vi "Main.vi"(11 "Module Admin":refnum<class "Delacor_lib_QMH_Module Admin.lvclass">) -> ()   [LabVIEW 2019, in "UI.lvlib"]
doc: "This template is based off of the Queued Message Handler design pattern and the Queued Message Handler project template that ships with LabVIEW.\n\nThe main difference is that the queue is private to this module and communication between modules is performed via Broadcast and Request events.\n\nRequest events are wrapped in public API methods and are handled in the Event Handling Loop (EHL) of this VI. Any module can register for Broadcast events sent by this module. The EHL generates messages based on user interface actions.\n\nThe Message Handling Loop (MHL) processes messages generated by the EHL, or by other messages. The messages are string values, so new messages can be added easily to the Message Cases case structure in the MHL. Each message cluster can also provide an optional value for Message Data, which is a variant that can be converted to whatever message-specific data is required.\n_____\nBased on Delacor QMH Project Template 5.0.0.82."
uses:
  UI.lvlib
  <vilib>/Delacor/Delacor QMH/Libraries/Module Admin_class/Delacor_lib_QMH_Module Admin.lvclass
  Module Data--cluster.ctl
  Stop Argument--cluster.ctl
  <vilib>/Delacor/Delacor QMH/Libraries/Message Queue_class/Delacor_lib_QMH_Message Queue.lvclass/Delacor_lib_QMH_Message Queue.ctl
  <vilib>/Delacor/Delacor QMH/Libraries/Module Admin_class/Delacor_lib_QMH_Module Admin.lvclass/Delacor_lib_QMH_Module Admin.ctl
  <vilib>/Utility/miscctls.llb/LVPointTypeDef.ctl
  <vilib>/Delacor/Delacor QMH/Libraries/Message Queue_class/Delacor_lib_QMH_Enqueue Message (Single).vi
  <vilib>/Delacor/Delacor QMH/Libraries/Module Admin_class/Delacor_lib_QMH_Get External Launch.vi
  <vilib>/Utility/error.llb/Error Cluster From Error Code.vi
  <vilib>/ErrorRing/Error Ring.xnode
  <vilib>/Delacor/Delacor QMH/Libraries/Message Queue_class/Delacor_lib_QMH_Message Queue.lvclass
  LabVIEW Data/DQMH Module Templates/Source/Luis/Modulo w HL(with Helper Loop)/Modulo w HL(with Helper Loop).lvlib
panel:
  in  "Stop Acq":bool
  in  "Start Acq":bool
  out "error out":errorcluster
  out "Status":string
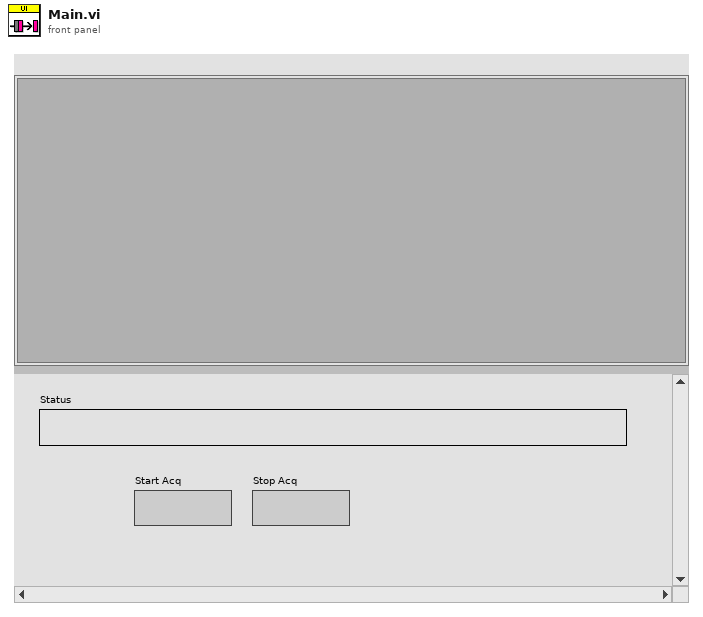
[diagram p1: front panel]
types:
  T1 = typedef "UI.lvlib/Request Events--cluster.ctl" = cluster{"Stop Module":refnum<user-event>, "Show Panel":refnum<user-event>, "Hide Panel":refnum<user-event>, "Get Module Execution Status":refnum<user-event>, "Show Diagram":refnum<user-event>}
  T2 = typedef "Aquisition.lvlib/Broadcast Events--cluster.ctl" = cluster{"Module Did Init":refnum<user-event>, "Status Updated":refnum<user-event>, "Error Reported":refnum<user-event>, "Module Did Stop":refnum<user-event>, "Update Module Execution Status":refnum<user-event>}
  T3 = typedef "UI.lvlib/Module Data--cluster.ctl" = cluster{"Status":string}
  T4 = enum32{"invalid lock state", "Not Locked", "Locked (No Password)", "Password-protected"}
  T5 = typedef "UI.lvlib/Stop Argument--cluster.ctl" = cluster{"Origin":string, "Exit via Stop Module Req?":bool, "Wait for Module to stop?":bool}
  T6 = enum32{"Invalid", "Standard", "Closed", "Hidden", "Minimized", "Maximized"}
  T7 = typedef "LVPointTypeDef.ctl" = cluster{"Horizontal":i16, "Vertical":i16}
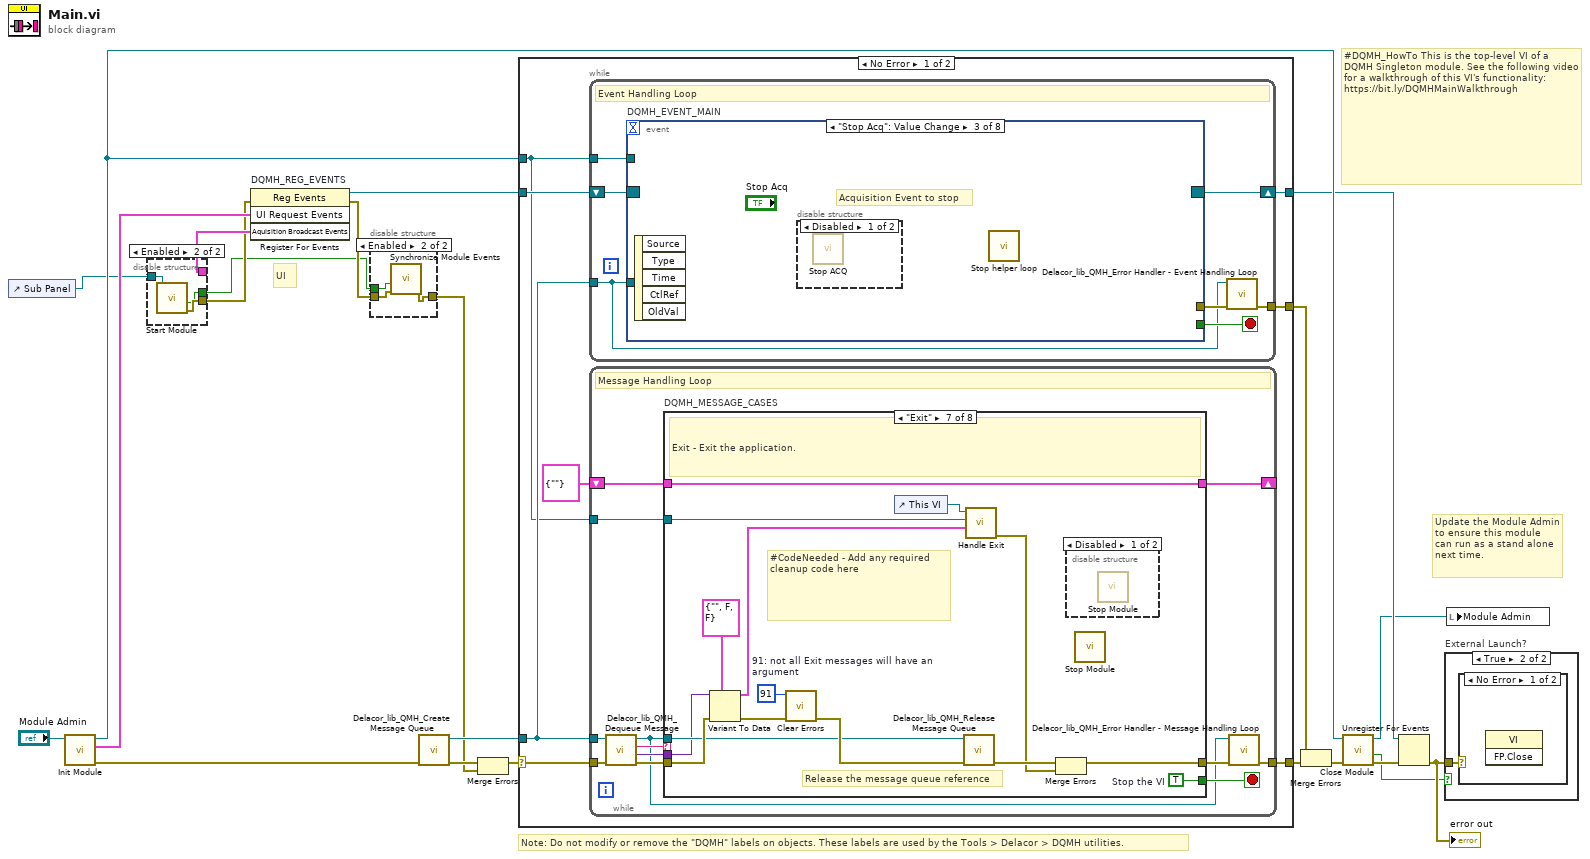
[diagram p0: block diagram]
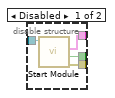
[diagram p2: hidden frame]
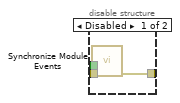
[diagram p3: hidden frame]
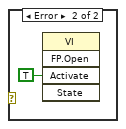
[diagram p5: hidden frame]
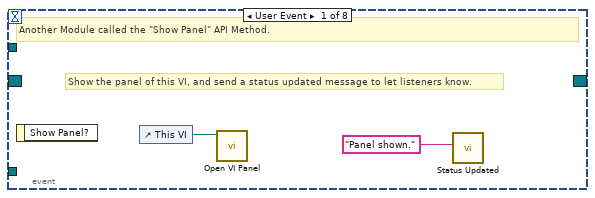
[diagram p6: hidden frame]
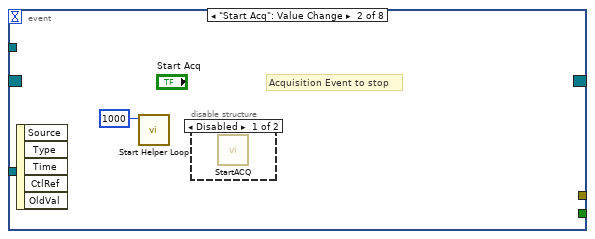
[diagram p7: hidden frame]
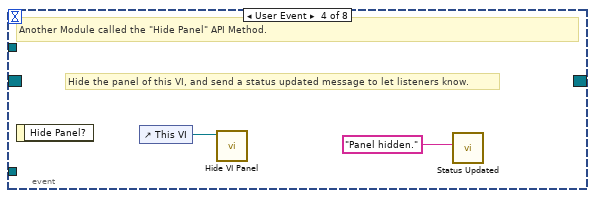
[diagram p10: hidden frame]
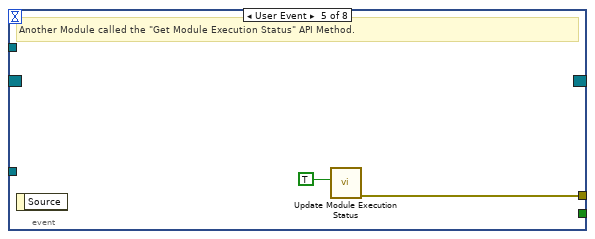
[diagram p11: hidden frame]
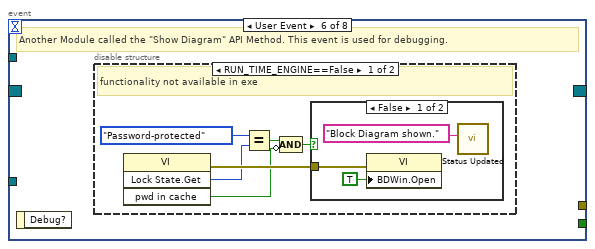
[diagram p12: hidden frame]
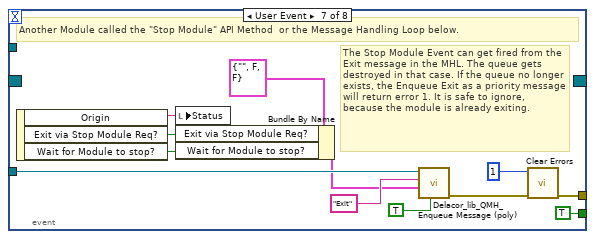
[diagram p15: hidden frame]
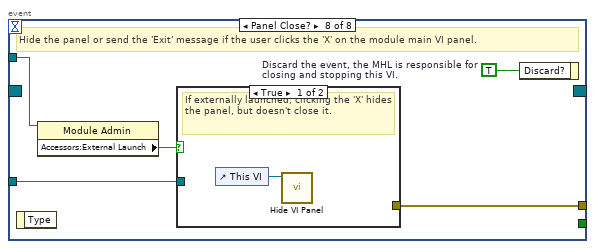
[diagram p16: hidden frame]
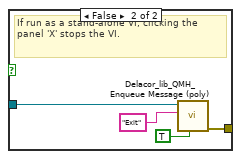
[diagram p17: hidden frame]
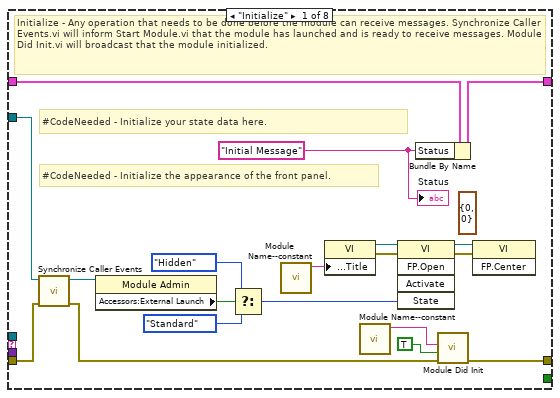
[diagram p18: hidden frame]
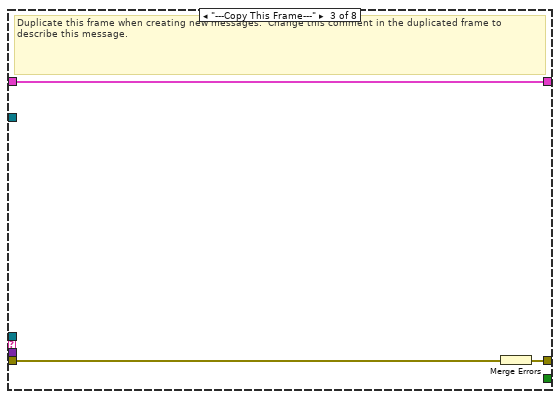
[diagram p20: hidden frame]
diagram:
  # "UI"
  # "#DQMH_HowTo This is the top-level VI of a DQMH Singleton module. See the following video for a walkthrough of this VI's functionality: https://bit.ly/DQMHMainWalkthrough"
  # "Note: Do not modify or remove the \"DQMH\" labels on objects. These labels are used by the Tools > Delacor > DQMH utilities."
  # "Update the Module Admin to ensure this module can run as a stand alone next time."
  n1 = control-ref of="Sub Panel"() -> (w1:refnum<vi>)
  n2 = call "Init Module.vi"("Singleton Module Admin in"="Module Admin") -> ("error out"=w21:errorcluster, "UI Request Events"=w11:T1, "Singleton Module Admin out"=w14:refnum<class "Delacor_lib_QMH_Module Admin.lvclass">)  [unwired: 8 in]
  n3 = disable-structure shown="Enabled" {
    disable-tunnel: [w26 _] -> w6
    disable-tunnel: [w25 w28] -> w5
    disable-tunnel: [w24 w27] -> w3
    disable-tunnel: w1 -> [w23 w29]
    frame Disabled {
      n4 = call "Start Module.vi"("ACQ Panel"=w23) -> ("error out"=w25:errorcluster, "Wait for Event Sync?"=w24:bool, "Aquisition Broadcast Events"=w26:T2)  [unwired: 7 in, 1 out]
    }
    frame Enabled {
      n5 = call "Start Module.vi"("Sub Panel"=w29) -> ("error out"=w28:errorcluster, "Wait for Event Sync?"=w27:bool)  [unwired: 7 in, 2 out]
    }
  }
  n6 = register-events "DQMH_REG_EVENTS"(error in=w5, w11, w6) -> (reference out=w12:refnum<event-registration>, error out=w4:errorcluster)  [unwired: 1 in]
  n7 = disable-structure shown="Enabled" {
    disable-tunnel: w4 -> [w32 w35]
    disable-tunnel: w3 -> [w31 w34]
    disable-tunnel: [w30 w33] -> w2
    frame Disabled {
      n8 = call "Synchronize Module Events.vi"("error in (no error)"=w32, "Wait for Event Sync?"=w31) -> ("error out"=w30:errorcluster)  [unwired: 9 in]
    }
    frame Enabled {
      n9 = call "Synchronize Module Events.vi"("error in (no error)"=w35, "Wait for Event Sync?"=w34) -> ("error out"=w33:errorcluster)  [unwired: 9 in]
    }
  }
  n10 = call <vilib>:"Delacor_lib_QMH_Create Message Queue.vi"("error in (no error)"=w21) -> ("error out"=w16:errorcluster, "Message Queue"=w10:refnum<class "Delacor_lib_QMH_Message Queue.lvclass">)  [unwired: 9 in]
  n11 = Merge Errors(w16, w2) -> (w15:errorcluster)
  n12 = case shown="No Error" w15 {
    selector: w15 -> [w41 w187]
    tunnel: [w43 w186] -> w22
    tunnel: [w40 w192] -> w13
    tunnel: w12 -> [w38 w192]
    tunnel: w10 -> [w37 w185]
    tunnel: [w42 _] -> w19
    tunnel: w14 -> [w36 w188]
    frame No Error {
      n13 = while {
        tunnel: w37 -> [w44]
        shift-right: [w47] -> w40
        shift-left: w38 -> [w48]
        tunnel: [w49] -> w42
        tunnel: w36 -> [w45]
        stop <- w46 stop-if-true
        # "Event Handling Loop"
        n14 = event "DQMH_EVENT_MAIN" shown="[2] \"Stop Acq\": Value Change" {
          selector: w48 -> [_ _ _ _ _ _ _ _]
          dyn-events: [_ _ _ _ _ _ _ _] -> w47
          timeout: _ -> [_ _ _ _ _ _ _ _]
          tunnel: [_ _ _ _ _ _ TRUE ("Discard?") _] -> w46
          tunnel: w44 -> [_ _ _ _ _ _ w74 w81]
          tunnel: [_ _ _ _ w57 _ w77 w83] -> w50
          tunnel: w45 -> [_ _ _ _ _ _ _ w80]
          event User Event {
            # "Show the panel of this VI, and send a status updated message to let listeners know."
            # "Another Module called the \"Show Panel\" API Method."
            n15 = event-data() -> ()  [unwired: 1 in, 1 out]
            n16 = control-ref of="This VI"() -> (w52:refnum<vi>)
            n17 = call "Open VI Panel.vi"("VI"=w52) -> ()  [unwired: 10 in, 1 out]
            n18 = call "Status Updated.vi"("Status"="Panel shown." ("format string")) -> ()  [unwired: 10 in, 1 out]
          }
          event "Start Acq": Value Change {
            # "Acquisition Event to stop"
            n19 = event-data() -> ()  [unwired: 1 in, 5 out]
            n20 = call "Start Helper Loop.vi"("Delay Timeout"=1000) -> ()  [unwired: 10 in, 1 out]
            n21 = disable-structure shown="Disabled" {
              frame Disabled {
                n22 = call "StartACQ.vi"() -> ()  [unwired: 11 in, 1 out]
              }
              frame Enabled {
              }
            }
          }
          event "Stop Acq": Value Change {
            # "Acquisition Event to stop"
            n23 = event-data() -> ()  [unwired: 1 in, 5 out]
            n24 = disable-structure shown="Disabled" {
              frame Disabled {
                n25 = call "Stop ACQ.vi"() -> ()  [unwired: 11 in, 1 out]
              }
              frame Enabled {
              }
            }
            n26 = call "Stop helper loop.vi"() -> ()  [unwired: 11 in, 1 out]
          }
          event User Event {
            # "Hide the panel of this VI, and send a status updated message to let listeners know."
            # "Another Module called the \"Hide Panel\" API Method."
            n27 = event-data() -> ()  [unwired: 1 in, 1 out]
            n28 = control-ref of="This VI"() -> (w55:refnum<vi>)
            n29 = call "Hide VI Panel.vi"("VI"=w55) -> ()  [unwired: 10 in, 1 out]
            n30 = call "Status Updated.vi"("Status"="Panel hidden." ("format string")) -> ()  [unwired: 10 in, 1 out]
          }
          event User Event {
            # "Another Module called the \"Get Module Execution Status\" API Method."
            n31 = event-data() -> ()  [unwired: 1 in, 1 out]
            n32 = call "Update Module Execution Status.vi"("Running?"=TRUE) -> ("error out"=w57:errorcluster)  [unwired: 10 in]
          }
          event User Event {
            # "Another Module called the \"Show Diagram\" API Method. This event is used for debugging."
            n33 = event-data() -> ()  [unwired: 1 in, 1 out]
            n34 = disable-structure shown="RUN_TIME_ENGINE==False" {
              frame condition #0 (active) {
                # "functionality not available in exe"
                n35 = invoke class="VI" method="Lock State.Get"() -> (error out=w63:errorcluster, "Get Lock State"=w62:T4, "pwd in cache"=w59:bool)  [unwired: 4 in, 1 out]
                n36 = Equal?(x=T4."Password-protected", y=w62) -> (x = y?=w60:bool)
                n37 = Compound Arithmetic op=AND(w60, invert w59) -> (w58:bool)
                n38 = case shown="False" w58 {
                  tunnel: w63 -> [w66 _]
                  frame False {
                    n39 = property class="VI"(error in=w66, "BDWin.Open"=TRUE ("Block Diagram Window:Open")) -> ()  [unwired: 1 in, 2 out]
                    n40 = call "Status Updated.vi"("Status"="Block Diagram shown." ("format string")) -> ()  [unwired: 10 in, 1 out]
                  }
                  frame True {
                    # "Password-protected VI, and the password is not in the cache. Do not show the diagram."
                  }
                }
              }
              frame condition #1 {
              }
            }
          }
          event User Event {
            # "The Stop Module Event can get fired from the Exit message in the MHL. The queue gets destroyed in that case. If the queue no longer exists, the Enqueue Exit as a priority message will return error 1. It is safe to ignore, because the module is already exiting."
            # "Another Module called the \"Stop Module\" API Method  or the Message Handling Loop below."
            n41 = event-data() -> ("Origin"=w73:string, "Exit via Stop Module Req?"=w69:bool, "Wait for Module to stop?"=w68:bool)  [unwired: 1 in]
            n42 = local write "Status"(w73) -> ()
            n43 = Bundle By Name(cluster=T5 {"Origin"="", "Exit via Stop Module Req?"=FALSE, "Wait for Module to stop?"=FALSE} ("Stop Argument"), "Exit via Stop Module Req?"=w69, "Wait for Module to stop?"=w68) -> (w67:T5)
            n44 = call-poly <vilib>:"Delacor_lib_QMH_Enqueue Message (poly).vi"("Priority Message? (F)"=TRUE, "Message Data"=w67, "Message"="Exit", "Message Queue in"=w74) -> ("error out"=w78:errorcluster)  [unwired: 6 in, 1 out]
            n45 = call <vilib>:"Clear Errors.vi"("error in (no error)"=w78, "specific error code to clear (0: all)"=1) -> ("error out"=w77:errorcluster)  [unwired: 4 in, 1 out]
          }
          event Panel Close? {
            w82 = TRUE  # Discard the event, the MHL is responsible for closing and stopping this VI.
            # "Hide the panel or send the 'Exit' message if the user clicks the 'X' on the module main VI panel."
            n46 = event-data() -> ()  [unwired: 1 in, 1 out]
            n47 = property class="Module Admin"(reference=w80) -> ("Accessors:External Launch"=w79:bool)  [unwired: 1 in, 2 out]
            n48 = case shown="True" w79 {
              tunnel: w81 -> [_ w87]
              tunnel: [_ w88] -> w83
              frame True {
                # "If externally launched, clicking the 'X' hides the panel, but doesn't close it."
                n49 = control-ref of="This VI"() -> (w84:refnum<vi>)
                n50 = call "Hide VI Panel.vi"("VI"=w84) -> ()  [unwired: 10 in, 1 out]
              }
              frame False {
                # "If run as a stand-alone VI, clicking the panel 'X' stops the VI."
                n51 = call-poly <vilib>:"Delacor_lib_QMH_Enqueue Message (poly).vi"("Priority Message? (F)"=TRUE, "Message"="Exit", "Message Queue in"=w87) -> ("error out"=w88:errorcluster)  [unwired: 7 in, 1 out]
              }
            }
            n52 = event-data("Discard?"=w82) -> ()  [unwired: 1 in, 1 out]
          }
        }
        n53 = call-dynamic "Delacor_lib_QMH_Error Handler - Event Handling Loop.vi"("error in (no error)"=w50, "Message Queue in"=w44) -> ("dup error in"=w49:errorcluster)  [unwired: 8 in, 1 out]
      }
      n54 = while {
        tunnel: w37 -> [w91]
        shift-right: [w95] -> _
        shift-left: T3 {"Status"=""} ("Data Cluster") -> [w96]
        tunnel: w41 -> [w99]
        tunnel: [w97] -> w43
        tunnel: w36 -> [w89]
        stop <- w94 stop-if-true
        # "Message Handling Loop"
        n55 = call-dynamic "Delacor_lib_QMH_Dequeue Message.vi"("error in (no error)"=w99, "Message Queue in"=w91) -> ("error out"=w98:errorcluster, "Message Data"=w92:variant, "Message"=w93:string, "Message Queue out"=w90:refnum<class "Delacor_lib_QMH_Message Queue.lvclass">)  [unwired: 6 in]
        n56 = case "DQMH_MESSAGE_CASES" shown="\"Exit\"" w93 {
          selector: w93 -> [_ _ _ _ _ _ _ w172]
          tunnel: w90 -> [_ _ _ _ _ w142 w164 _]
          tunnel: w98 -> [w117 w121 w124 w126 w131 w149 w170 w174]
          tunnel: [w115 w121 w123 w126 w130 w145 w167 w175] -> w100
          tunnel: w96 -> [w106 w120 w122 w125 w128 w144 w163 w173]
          tunnel: [w105 w120 w122 w125 w128 w144 w163 w173] -> w95
          tunnel: [_ _ _ _ _ _ w162 _] -> w94
          tunnel: w92 -> [_ _ _ _ _ w143 w161 _]
          tunnel: w89 -> [w107 _ _ _ _ w141 w156 _]
          frame "Initialize" {
            (unwired) T7 {"Horizontal"=0, "Vertical"=0} ("Origin")
            w101 = "Initial Message" ("Initial Message")
            # "#CodeNeeded - Initialize the appearance of the front panel."
            # "#CodeNeeded - Initialize your state data here."
            # "Initialize - Any operation that needs to be done before the module can receive messages. Synchronize Caller Events.vi will inform Start Module.vi that the module has launched and is ready to receive messages. Module Did Init.vi will broadcast that the module initialized."
            n57 = call "Synchronize Caller Events.vi"("error in (no error)"=w117, "Singleton Module Admin in"=w107) -> ("error out"=w116:errorcluster, "Singleton Module Admin out"=w102:refnum<class "Delacor_lib_QMH_Module Admin.lvclass">)  [unwired: 8 in]
            n58 = property class="Module Admin"(reference=w102) -> ("Accessors:External Launch"=w111:bool)  [unwired: 1 in, 2 out]
            n59 = Select(t=T6."Hidden" ("State"), s=w111, f=T6."Standard" ("State")) -> (s? t:f=w108:T6)
            n60 = call "Module Name--constant.vi"() -> ("Module Name"=w114:string)  [unwired: 11 in]
            n61 = property class="VI"("Front Panel.Title"=w114) -> (reference out=w113:refnum<vi>, error out=w119:errorcluster)  [unwired: 2 in]
            n62 = call "Module Name--constant.vi"() -> ("Module Name"=w103:string)  [unwired: 11 in]
            n63 = invoke class="VI" method="FP.Open"(reference=w113, error in=w119, "State"=w108) -> (reference out=w112:refnum<vi>, error out=w118:errorcluster)  [unwired: 2 in, 3 out]
            n64 = Bundle By Name(cluster=w106, "Status"=w101) -> (w105:T3)
            n65 = call "Module Did Init.vi"("error in (no error)"=w116, "Initialized?"=TRUE, "Origin"=w103) -> ("error out"=w115:errorcluster)  [unwired: 8 in]
            n66 = invoke class="VI" method="FP.Center"(reference=w112, error in=w118) -> ()  [unwired: 1 in, 3 out]
            "Status" <- w101
          }
          frame "--- Module Specific ---" {
            # "Separator -- The following cases handle messages specific to this Module."
          }
          frame "---Copy This Frame---" {
            # "Duplicate this frame when creating new messages.  Change this comment in the duplicated frame to describe this message."
            n67 = Merge Errors(w124) -> (w123:errorcluster)
          }
          frame "--- Exit and Error Handling---" {
            # "Separator - The following cases handle errors and exit messages."
          }
          frame "Simulate MHL Error" {
            # "#DQMH_HowTo The 'Simulate MHL Error' button  illustrates how the MHL handles errors. This event is instructional in nature and can be removed."
            # "Simulate an error occurring at the MHL"
            n68 = call "Module Name--constant.vi"() -> ("Module Name"=w127:string)  [unwired: 11 in]
            n69 = xnode "Error Ring"("parameter 0"=w127) -> ("error out"=w129:errorcluster)
            n70 = Merge Errors(w131, w129) -> (w130:errorcluster)
          }
          frame "Error" {
            # "#CodeRecommended - If you ever change the name of this \"Error\" message, you'll need to update the name in the Check Loop Error.vi as well."
            # "#CodeRecommended - If the module is running in standalone mode (External Launch = FALSE), this code will pop up an error dialog and call the 'Exit' message if an error occurs. Add more fine-grained error handling here."
            # "Error - Check the error message data and respond accordingly. This message is sent by the \"Error Handler\" VIs at the end of each loop in this application."
            n71 = property class="Module Admin"(reference=w141) -> ("Accessors:External Launch"=w140:bool)  [unwired: 1 in, 2 out]
            n72 = Variant To Data(error in=w149, type=errorcluster {"status"=FALSE, "code"=0, "source"=""} ("error constant"), Variant=w143) -> (data=w150:errorcluster, error out=w147:errorcluster)
            n73 = call "Module Name--constant.vi"() -> ("Module Name"=w139:string)  [unwired: 11 in]
            n74 = call "Error Reported.vi"("Additional Information"=w139, "Error"=w150) -> ()  [unwired: 9 in, 1 out]
            n75 = case shown="False" w140 {
              tunnel: [w155 _] -> w146
              tunnel: w142 -> [w153 _]
              tunnel: w150 -> [w154 _]
              frame False {
                # "If the module is running standalone, then pop up an error dialog and call the \"Exit\" message."
                n76 = call <vilib>:"Simple Error Handler.vi"("error in (no error)"=w154) -> ()  [unwired: 4 in, 5 out]
                n77 = call-poly <vilib>:"Delacor_lib_QMH_Enqueue Message (poly).vi"("Priority Message? (F)"=TRUE, "Message"="Exit", "Message Queue in"=w153) -> ("error out"=w155:errorcluster)  [unwired: 7 in, 1 out]
              }
              frame True {
                # "If the module was launched externally, calling the Error Reported broadcast VI is the only action performed by the \"Error\" message. The module's caller can then process the error appropriately."
              }
            }
            n78 = Merge Errors(w147, w146) -> (w145:errorcluster)
            n79 = local write "error out"(w145) -> ()
          }
          frame "Exit" {
            w160 = 91  # 91: not all Exit messages will have an argument
            w162 = TRUE  # Stop the VI
            # "Release the message queue reference"
            # "#CodeNeeded - Add any required cleanup code here"
            # "Exit - Exit the application."
            n80 = Variant To Data(error in=w170, type=T5 {"Origin"="", "Exit via Stop Module Req?"=FALSE, "Wait for Module to stop?"=FALSE} ("Stop Argument"), Variant=w161) -> (data=w158:T5, error out=w166:errorcluster)
            n81 = call <vilib>:"Clear Errors.vi"("error in (no error)"=w166, "specific error code to clear (0: all)"=w160) -> ("error out"=w169:errorcluster)  [unwired: 4 in, 1 out]
            n82 = control-ref of="This VI"() -> (w157:refnum<vi>)
            n83 = call-dynamic "Delacor_lib_QMH_Release Message Queue.vi"("error in (no error)"=w169, "Message Queue"=w164) -> ("error out"=w168:errorcluster)  [unwired: 9 in]
            n84 = call "Handle Exit.vi"("Stop Argument"=w158, "Admin in"=w156, "VI reference"=w157) -> ("error out"=w165:errorcluster)  [unwired: 7 in, 1 out]
            n85 = Merge Errors(w168, w165) -> (w167:errorcluster)
            n86 = disable-structure shown="Disabled" {
              frame Disabled {
                n87 = call "Stop Module.vi"() -> ()  [unwired: 11 in, 1 out]
              }
              frame Enabled {
              }
            }
            n88 = call "Stop Module.vi"() -> ()  [unwired: 11 in, 1 out]
          }
          frame Default {
            # "'Default' case only runs if there is a message that isn't defined in any of the other cases.  Output a programming error."
            n89 = call "Module Name--constant.vi"() -> ("Module Name"=w171:string)  [unwired: 11 in]
            n90 = xnode "Error Ring"("parameter 0"=w172, "parameter 1"=w171) -> ("error out"=w176:errorcluster)
            n91 = Merge Errors(w174, w176) -> (w175:errorcluster)
          }
        }
        n92 = call-dynamic "Delacor_lib_QMH_Error Handler - Message Handling Loop.vi"("error in (no error)"=w100, "Message Queue in"=w90) -> ("dup error in"=w97:errorcluster)  [unwired: 8 in, 1 out]
      }
    }
    frame Error {
      # "Synchronize Caller Events.vi will inform Start Module.vi that the module has launched and will let the code calling Start Module.vi register for broadcasts and would permit the caller receive the broadcast that an error occurred at launch time."
      n93 = call-dynamic "Delacor_lib_QMH_Release Message Queue.vi"("error in (no error)"=w187, "Message Queue"=w185) -> ("error out"=w186:errorcluster)  [unwired: 9 in]
      n94 = call "Synchronize Caller Events.vi"("Singleton Module Admin in"=w188) -> ("error out"=w193:errorcluster)  [unwired: 9 in, 1 out]
      n95 = call "Module Name--constant.vi"() -> ("Module Name"=w191:string)  [unwired: 11 in]
      n96 = Format Into String(format string="An error occurred during initialization. %s is no longer running.", w191) -> (resulting string=w189:string)  [unwired: 2 in, 1 out]
      n97 = Merge Errors(w186, w193) -> (w194:errorcluster)
      n98 = call "Error Reported.vi"("Additional Information"=w189, "Error"=w194) -> ()  [unwired: 9 in, 1 out]
    }
  }
  n99 = Merge Errors(w19, w22) -> (w18:errorcluster)
  n100 = call "Close Module.vi"("error in (no error)"=w18, "Module Admin in"=w14) -> ("error out"=w20:errorcluster, "External Launch"=w7:bool, "Module Admin out"=w8:refnum<class "Delacor_lib_QMH_Module Admin.lvclass">)  [unwired: 7 in]
  n101 = Unregister For Events(event registration refnum=w13, error in=w20) -> (error out=w17:errorcluster)
  "error out" <- w17
  n102 = case "External Launch?" shown="True" w7 {
    tunnel: w17 -> [_ w195]
    frame False {
    }
    frame True {
      n103 = case shown="No Error" w195 {
        frame No Error {
          n104 = invoke class="VI" method="FP.Close"() -> ()  [unwired: 3 in, 3 out]
        }
        frame Error {
          n105 = invoke class="VI" method="FP.Open"("Activate"=TRUE ("Activate?")) -> ()  [unwired: 4 in, 5 out]
        }
      }
    }
  }
  n106 = local write "Module Admin"(w8) -> ()
